vi "Memory.Pointer.Advanced Copy.Adjust Parameters.vi"(5 "host byte order (little-endian)":enum16{"big-endian", "little-endian"}(ring)=enum."little-endian", 7 "target byte order (big-endian)":enum16{"big-endian", "little-endian"}(ring), 8 "dst width":u64 format="%d bytes", 9 "src width":u64 format="%d bytes", 10 "dst offset in":u64 format="%d bytes", 11 "src offset in":u64 format="%d bytes") -> (0 "bytes to move":u64, 1 "dst clear size":u64, 2 "dst offset out":u64 format="%d bytes", 3 "src offset out":u64 format="%d bytes")   [LabVIEW 2016, in "Memory Manager.lvlib" / "Memory.Pointer.lvclass"]
uses:
  Memory.Pointer.lvclass
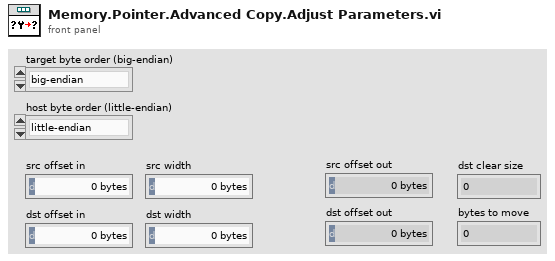
[diagram p1: front panel]
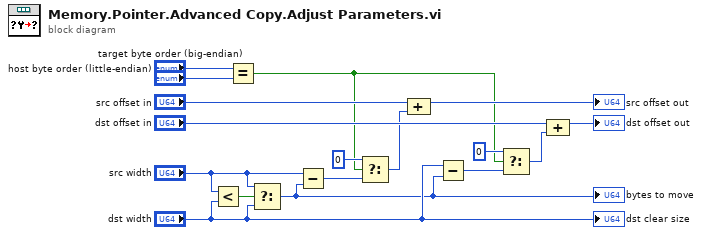
[diagram p0: block diagram]
diagram:
  n1 = Less?(x="src width", y="dst width") -> (x < y?=w15:bool)
  n2 = Equal?(x="host byte order (little-endian)", y="target byte order (big-endian)") -> (x = y?=w1:bool)
  n3 = Select(t="src width", s=w15, f="dst width") -> (s? t:f=w10:u64)
  "bytes to move" <- w10
  n4 = Subtract(x="src width", y=w10) -> (x-y=w7:u64)
  n5 = Select(t=u64 0, s=w1, f=w7) -> (s? t:f=w6:u64)
  n6 = Compound Arithmetic op=ADD("src offset in", w6) -> (→"src offset out":u64)
  n7 = Subtract(x="dst width", y=w10) -> (x-y=w4:u64)
  n8 = Select(t=u64 0, s=w1, f=w4) -> (s? t:f=w3:u64)
  n9 = Compound Arithmetic op=ADD("dst offset in", w3) -> (→"dst offset out":u64)
  "dst clear size" <- "dst width"
